vi "Config.vi"(8 "error in (no error)":errorcluster, 10 "Digital Configuration":T1) -> (0 "error out":errorcluster, 3 "Mech Pump out":refnum<class "Mech Pump.lvclass">)   [LabVIEW 2021, in "Mech Pump.lvlib" / "Mech Pump.lvclass"]
uses:
  Mech Pump.lvclass
  Mech Pump.lvclass/Mech Pump.ctl
  DAQ-arch/Digital Configure.ctl
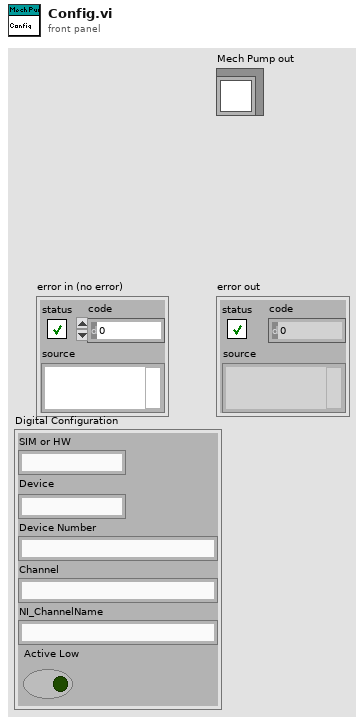
[diagram p1: front panel]
types:
  T1 = typedef "Digital Configure.ctl" = cluster{"SIM or HW":string, "Device":string, "Device Number":string, "Channel":string, "NI_ChannelName":string, "Active Low":bool}
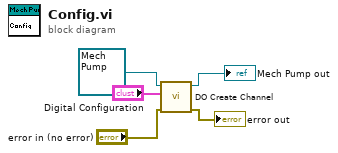
[diagram p0: block diagram]
diagram:
  n1 = call "DO Create Channel.vi"("error in (no error)"="error in (no error)", "Digital Configuration"="Digital Configuration", "Mech Pump in"=refnum<class "Mech Pump.lvclass"> refnum) -> ("error out"=→"error out":errorcluster, "Mech Pump out"=→"Mech Pump out":refnum<class "Mech Pump.lvclass">)  [unwired: 7 in]
